vi "Aim Angle for Drive.vi"   [LabVIEW 2016]
types:
  T1 = typedef "Command Status Info.ctl" = cluster{"Name":string, "Status":T2, "notifier out":T3}
  T2 = typedef "Completion Status.ctl" = enum16{"Successful", "Aborted", "Incomplete"}
  T3 = typedef "Completion Notifier.ctl" = refnum<notifier>
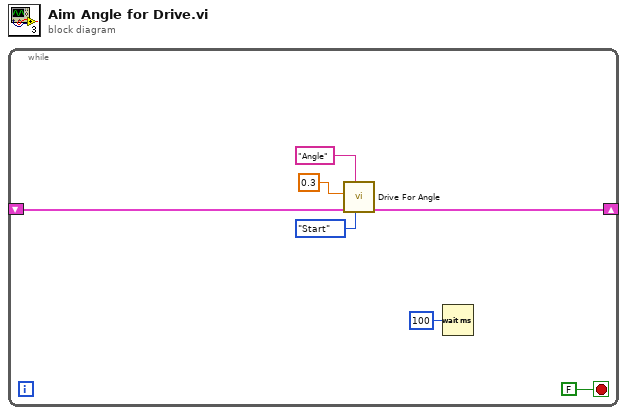
[diagram p0: block diagram]
diagram:
  n1 = while {
    shift-right: [w1] -> _
    shift-left: _ -> [w2]
    stop <- FALSE stop-if-true
    n2 = call "Drive For Angle.vi"("Synchronization"=enum16{"Start", "Wait"}."Start", "Description"="Angle", "Command Info In"=w2, "Speed"=0.3) -> ("Command Info Out"=w1:T1)  [unwired: 6 in, 1 out]
    n3 = Wait (ms)(milliseconds to wait=u32 100) -> ()  [unwired: 1 out]
  }
